vi "Chamber IP Ping.vi"(8 "error in (no error)":errorcluster) -> (0 "error out":errorcluster, 2 "Report Text":string, 3 "Chamber IP Ping?":bool)   [LabVIEW 2023, in "LTT_TeststandSteptypes.lvlib"]
uses:
  LTT_TeststandSteptypes.lvlib
  HardwareAbstractionLayer_LVOOP/Database/Database.lvclass
  HardwareAbstractionLayer_LVOOP/Database/SQL Public VI/Control/DB Options.ctl
  <userlib>/_OpenG.lib/error/error.llb/openg_error.lvlib
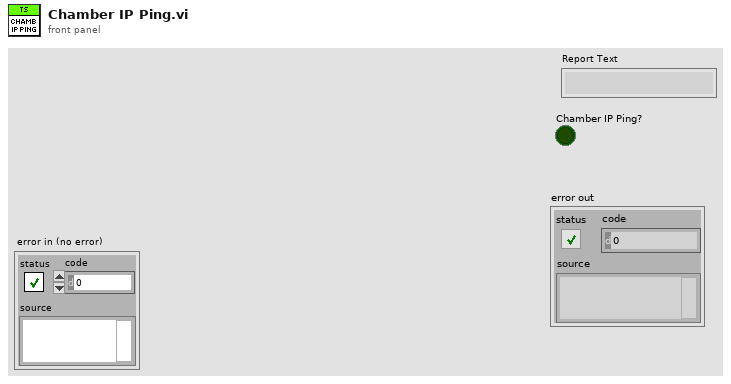
[diagram p1: front panel]
types:
  T1 = typedef "HardwareAbstractionLayer_LVOOP.lvlib/Database.lvclass/DB Options.ctl" = enum16{"Init", "Select Data", "Insert Data", "Update Data", "Delete Data", "Execute Query", "Create Schema", "Create Table", "List Tables", "List Columns", "Close"}
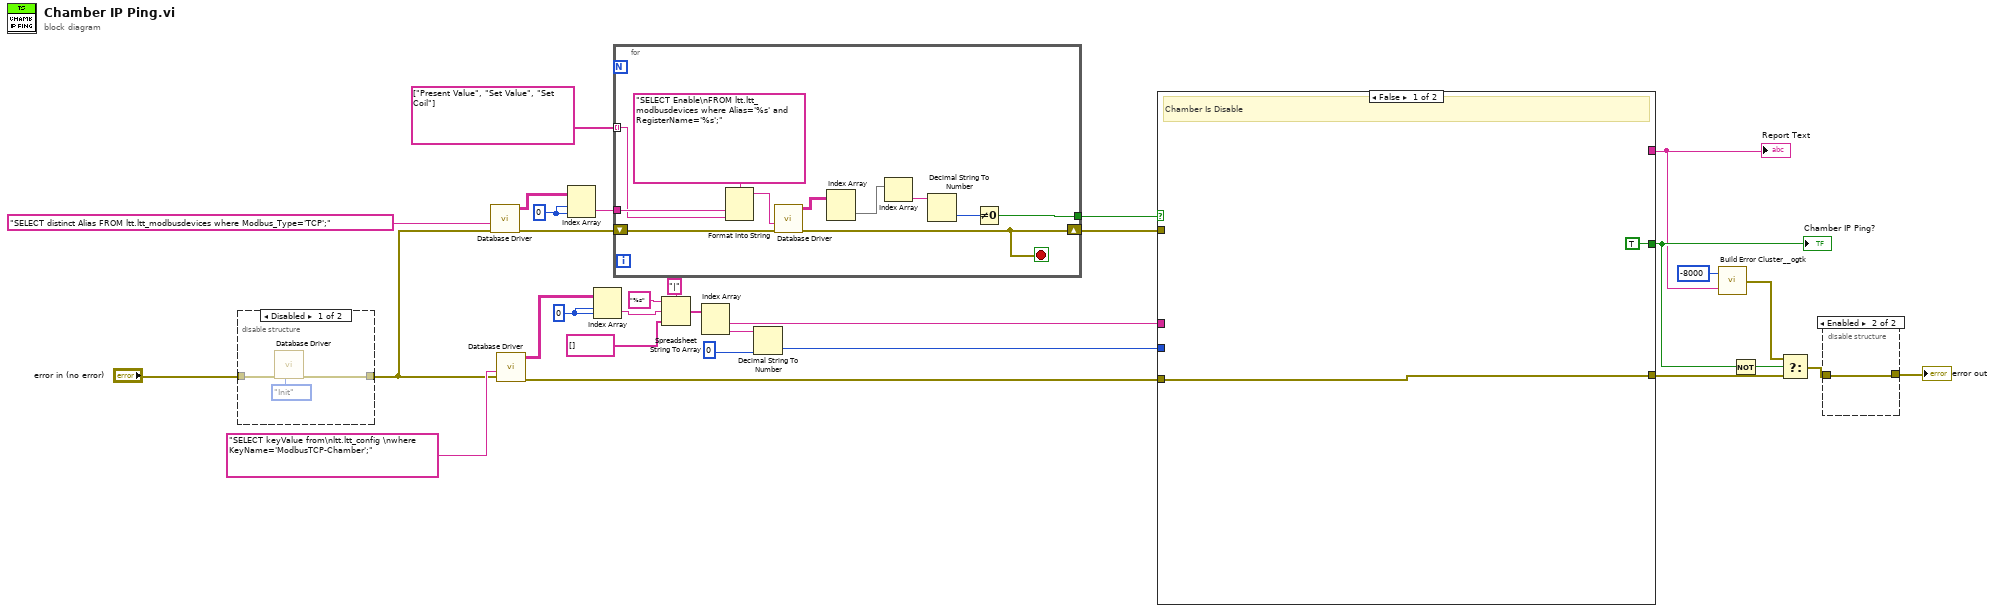
[diagram p0: block diagram]
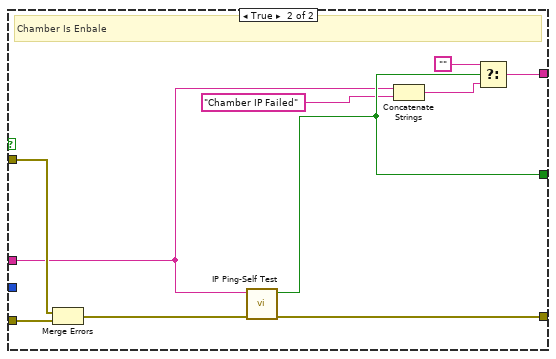
[diagram p2: hidden frame]
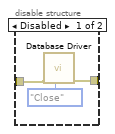
[diagram p4: hidden frame]
diagram:
  w16 = 0 ("disabled index (col)")
  w24 = 0 ("index (row)")
  n1 = disable-structure shown="Disabled" {
    disable-tunnel: "error in (no error)" -> [w33 w35]
    disable-tunnel: [w32 w35] -> w8
    frame Disabled {
      n2 = call "Database Driver.vi"("Options"=DB_Options."Init", "error in"=w33) -> ("error out"=w32:errorcluster)  [unwired: 6 in, 3 out]
    }
    frame Enabled {
    }
  }
  n3 = call "Database Driver.vi"("error in"=w8, "SQL query"="SELECT distinct Alias FROM ltt.ltt_modbusdevices where Modbus_Type='TCP';") -> ("error out"=w15:errorcluster, "data"=w17:string[][])  [unwired: 6 in, 2 out]
  n4 = call "Database Driver.vi"("error in"=w8, "SQL query"="SELECT keyValue from\nltt.ltt_config \nwhere KeyName='ModbusTCP-Chamber';") -> ("error out"=w19:errorcluster, "data"=w25:string[][])  [unwired: 6 in, 2 out]
  n5 = Index Array(array=w17, index (row)=w16, index (col)=w16) -> (element=w18:string)
  n6 = Index Array(array=w25, index (row)=w24, index (col)=w24) -> (element=w31:string)
  n7 = for {
    tunnel: w18 -> [w40]
    shift-right: [w42] -> w13
    shift-left: w15 -> [w41]
    tunnel: string[] ["Present Value", "Set Value", "Set Coil"] -> [w39] mode=indexing
    tunnel: [w36] -> w9
    stop <- w42 stop-if-true
    n8 = Format Into String(format string="SELECT Enable\nFROM ltt.ltt_modbusdevices where Alias='%s' and RegisterName='%s';", w40, w39) -> (resulting string=w46:string)  [unwired: 2 in, 1 out]
    n9 = call "Database Driver.vi"("error in"=w41, "SQL query"=w46) -> ("error out"=w42:errorcluster, "data"=w45:string[][])  [unwired: 6 in, 2 out]
    n10 = Index Array(array=w45) -> (element=w44:string[])  [unwired: 2 in]
    n11 = Index Array(array=w44) -> (element=w38:string)  [unwired: 1 in]
    n12 = Decimal String To Number(string=w38) -> (number=w37:i32)  [unwired: 2 in, 1 out]
    n13 = Not Equal To 0?(x=w37) -> (x != 0?=w36:bool)
  }
  n14 = Spreadsheet String To Array(delimiter (Tab)="|" ("format string"), format string="%s", spreadsheet string=w31, array type (2D Dbl)=string[] []) -> (array=w29:string[])
  n15 = Index Array(array=w29) -> (element #1=w20:string, element #2=w22:string)  [unwired: 2 in]
  n16 = Decimal String To Number(string=w22, default (0L)=u16 0 ("Port")) -> (number=w21:u16)  [unwired: 1 in, 1 out]
  n17 = case shown="False" w9 {
    tunnel: w21 -> [_ _]
    tunnel: w20 -> [_ w52]
    tunnel: w19 -> [w48 w57]
    tunnel: w13 -> [_ w58]
    tunnel: [w48 w55] -> w4
    tunnel: [TRUE ("Sucessful?") w54] -> w5
    tunnel: [_ w50] -> w2
    frame False {
      # "Chamber Is Disable"
    }
    frame True {
      # "Chamber Is Enbale"
      n18 = Merge Errors(w58, w57) -> (w56:errorcluster)
      n19 = call "IP Ping-Self Test.vi"("error in (no error)"=w56, "IP/Address"=w52) -> ("error out"=w55:errorcluster, "Sucessful?"=w54:bool)  [unwired: 8 in]
      n20 = Concatenate Strings(w52, "Chamber IP Failed" ("string")) -> (w53:string)
      n21 = Select(t="", s=w54, f=w53) -> (s? t:f=w50:string)
    }
  }
  "Chamber IP Ping?" <- w5
  "Report Text" <- w2
  n22 = call <userlib>:"Build Error Cluster__ogtk.vi"("String to Prepend to source (\"\")"=w2, "code"=-8000) -> ("error out"=w7:errorcluster)
  n23 = Not(x=w5) -> (.not. x?=w1:bool)
  n24 = Select(t=w7, s=w1, f=w4) -> (s? t:f=w3:errorcluster)
  n25 = disable-structure shown="Enabled" {
    disable-tunnel: w3 -> [w60 w62]
    disable-tunnel: [w59 w62] -> w10
    frame Disabled {
      n26 = call "Database Driver.vi"("Options"=DB_Options."Close", "error in"=w60) -> ("error out"=w59:errorcluster)  [unwired: 6 in, 3 out]
    }
    frame Enabled {
    }
  }
  "error out" <- w10
